vi "Frame Counter.vi"(1 "Action":T1=enum."Plus One") -> (0 "Num":i32)   [LabVIEW 2014]
uses:
  Focus Lock/Controls/Counter Action.ctl
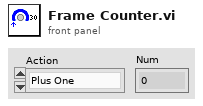
[diagram p1: front panel]
types:
  T1 = typedef "Counter Action.ctl" = enum16{"Zero", "Plus One", "Read"}
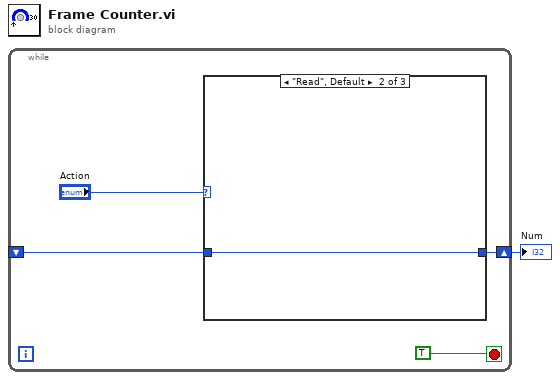
[diagram p0: block diagram]
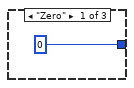
[diagram p2: hidden frame]
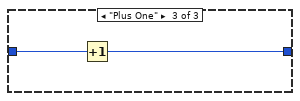
[diagram p3: hidden frame]
diagram:
  n1 = while {
    shift-right: [w4] -> w1
    shift-left: _ -> [w3]
    stop <- TRUE stop-if-true
    n2 = case shown="\"Read\", Default" "Action" {
      tunnel: [0 w7 w8] -> w4
      tunnel: w3 -> [_ w7 w9]
      frame "Zero" {
      }
      frame "Read", Default {
      }
      frame "Plus One" {
        n3 = Increment(x=w9) -> (x+1=w8:i32)
      }
    }
  }
  "Num" <- w1
